vi "Critical Priority.vi"() -> (3 "critical priority":i32=500)   [LabVIEW 2018, in "Dynamic Shared Variables.lvlib"]
doc: "The numerical threshold for critical alarm priorities. If the alarm priority is at or above this number, then the alarm is considered critical and will be red. Below this value, the alarm is non-critical and will be yellow."
uses:
  Dynamic Shared Variables.lvlib
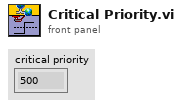
[diagram p1: front panel]
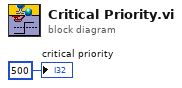
[diagram p0: block diagram]
diagram:
  "critical priority" <- 500
